vi "Start Key.vi"(8 "ErrorIn":errorcluster, 11 "VISAIn":refnum<visa-resource-name>) -> (0 "ErrorOut":errorcluster, 3 "VISAOut":refnum<visa-resource-name>)   [LabVIEW 2017, in "I28Drivers.lvlib"]
uses:
  I28Drivers.lvlib
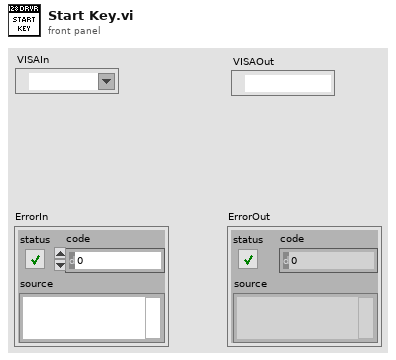
[diagram p1: front panel]
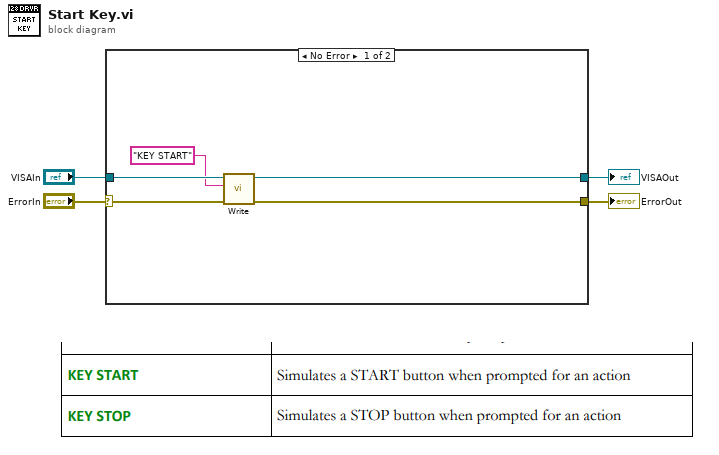
[diagram p0: block diagram]
diagram:
  n1 = case shown="No Error" "ErrorIn" {
    selector: "ErrorIn" -> [w9 w10]
    tunnel: "VISAIn" -> [w8 w11]
    tunnel: [w6 w11] -> w1
    tunnel: [w5 w10] -> w2
    frame No Error {
      n2 = call "Write.vi"("ErrorIn"=w9, "Command"="KEY START", "VISAIn"=w8) -> ("ErrorOut"=w5:errorcluster, "VISAOut"=w6:refnum<visa-resource-name>)  [unwired: 7 in]
    }
    frame Error {
    }
  }
  "ErrorOut" <- w2
  "VISAOut" <- w1
